vi "DataLog Tag Subset Last_srv.vi"(0 "subset indices":i32[](array[numeric]), 7 "certificate":string) -> (4 "values":dbl[](array[numeric]) format="%.2f", 8 "meta masks":u32[](array[numeric]) format="%.0b", 15 "error out":errorcluster)   [LabVIEW 2012]
doc: "This VI retrieves the last values of a subset of tags (as specified via an array of indices) from the memory buffers of the tags. In addition, the limit exceeded bit mask is retrieved from the tag meta tags object. This VI is intended for remote calling and serves to aggregate what would otherwise would be a series of subsequent VI server call into a single VI server call thereby minimizing network taxation. Using the returned results, a live display of tag values can be updated. Those tags that exceed limits can be coloured or otherwise flagged. Note that there is a very slight risk of a value and the corresponding mask being out of sync."
uses:
  clientsrv/typedefs/t_ClientSrv Access Levels.ctl
  typedefs/t_DataLog Tag Buffers Methods.ctl
  typedefs/t_DataLog Tag Meta Tags Methods.ctl
panel:
  # "Update panel typedef\nafter changing panel."
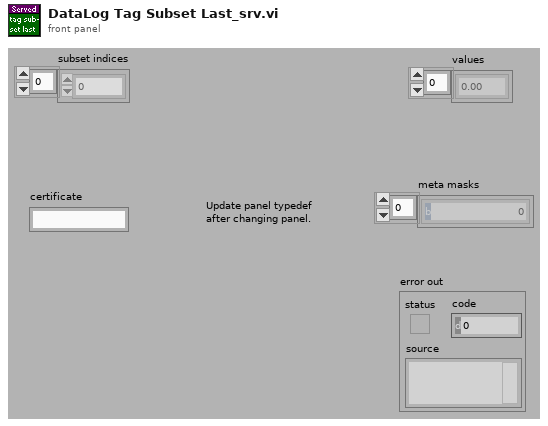
[diagram p1: front panel]
types:
  T1 = typedef "t_ClientSrv Access Levels.ctl" = enum16{"observer", "operator", "local"}
  T2 = typedef "t_DataLog Tag Meta Tags Methods.ctl" = enum16{"initialize", "apply and write", "get exceeded", "get metas", "cleanup"}
  T3 = typedef "t_DataLog Tag Buffers Methods.ctl" = enum16{"initialize", "inert", "write", "read", "read oldest", "read last", "cleanup"}
  T4 = typedef "t_DataLog Point.ctl" = cluster{"time":dbl, "value":dbl}
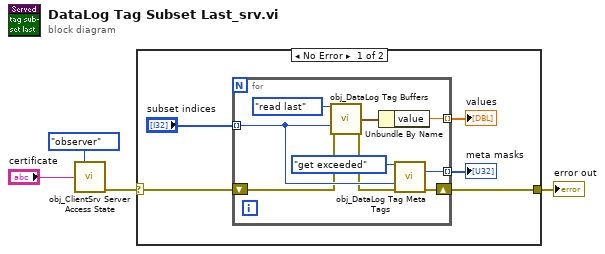
[diagram p0: block diagram]
diagram:
  n1 = call "obj_ClientSrv Server Access State.vi"("access level"=t_ClientSrv_Access_Levels."observer", "certificate in"="certificate") -> ("error out"=w3:errorcluster)  [unwired: 11 in, 2 out]
  n2 = case shown="No Error" w3 {
    selector: w3 -> [w5 w19]
    tunnel: [w6 w19] -> w4
    frame No Error {
      n3 = for {
        tunnel: "subset indices" -> [w15] mode=indexing
        tunnel: [w16] -> w8 mode=indexing
        tunnel: [w13] -> w7 mode=indexing
        shift-right: [w10] -> w6
        shift-left: w5 -> [w12]
        n4 = call "obj_DataLog Tag Buffers.vi"("method"=t_DataLog_Tag_Buffers_Methods."read last", "tag index"=w15, "error in (no error)"=w12) -> ("point out"=w17:T4, "error out"=w11:errorcluster)  [unwired: 8 in, 3 out]
        n5 = Unbundle By Name(w17) -> ("value"=w16:dbl)
        n6 = call "obj_DataLog Tag Meta Tags.vi"("method"=t_DataLog_Tag_Meta_Tags_Methods."get exceeded", "tag index in"=w15, "error in (no error)"=w11) -> ("exceeded mask"=w13:u32, "error out"=w10:errorcluster)  [unwired: 8 in, 3 out]
      }
      "values" <- w8
      "meta masks" <- w7
    }
    frame Error {
    }
  }
  "error out" <- w4
